vi "Checkers King Drawer.vi"() -> ()   [LabVIEW 2016]
panel:
  out "new picture":picture
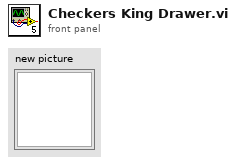
[diagram p1: front panel]
types:
  T1 = cluster{"Font Name:":string, "Size":i16, "Strikeout?":bool, "Italic?":bool, "Underline?":bool, "Outline?":bool, "Shadow?":bool, "Bold?":bool}
  T2 = cluster{"left":i16, "top":i16, "right":i16, "bottom":i16}
  T3 = enum16{"User-specified Font", "Application Font", "System Font", "Dialog Font"}
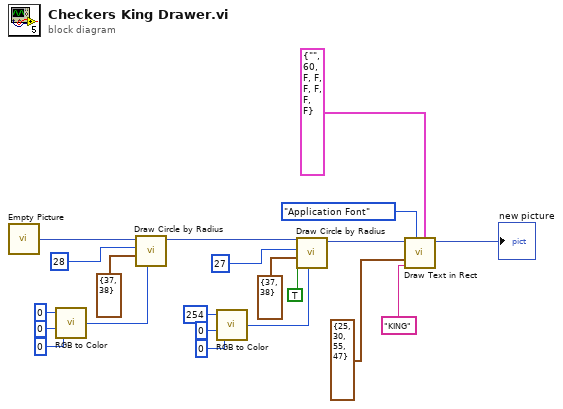
[diagram p0: block diagram]
diagram:
  n1 = call "Empty Picture"() -> ("empty picture"=w18:picture)
  n2 = call <vilib>:"RGB to Color.vi"("B"=u8 0, "G"=u8 0, "R"=u8 0) -> ("Color"=w21:u32)
  n3 = call <vilib>:"Draw Circle by Radius.vi"("color(black)"=w21, "pixel center"=cluster{"horizontal":i16, "vertical":i16} {"horizontal"=37, "vertical"=38}, "radius"=i16 28, "picture"=w18) -> ("new picture"=w8:picture)  [unwired: 7 in]
  n4 = call <vilib>:"RGB to Color.vi"("B"=u8 0, "G"=u8 0, "R"=u8 254) -> ("Color"=w9:u32)
  n5 = call <vilib>:"Draw Circle by Radius.vi"("color(black)"=w9, "fill?(F)"=TRUE, "pixel center"=cluster{"horizontal":i16, "vertical":i16} {"horizontal"=37, "vertical"=38}, "radius"=i16 27, "picture"=w8) -> ("new picture"=w6:picture)  [unwired: 6 in]
  n6 = call <vilib>:"Draw Text in Rect.vi"("[user-specified font]"=T1 {"Font Name:"="", "Size"=60, "Strikeout?"=FALSE, "Italic?"=FALSE, "Underline?"=FALSE, "Outline?"=FALSE, "Shadow?"=FALSE, "Bold?"=FALSE}, "desired font(Application)"=T3."Application Font", "text"="KING", "rect"=T2 {"left"=25, "top"=30, "right"=55, "bottom"=47}, "picture"=w6) -> ("new picture"=→"new picture":picture)  [unwired: 6 in]
